vi "基础23.vi"() -> ()   [LabVIEW 2014]
panel:
  out "簇 2":cluster{"数组":dbl[], "数组 2":dbl[]}
  in  "布尔":bool
  in  "簇":cluster{"数组":dbl[], "数组 2":dbl[]}
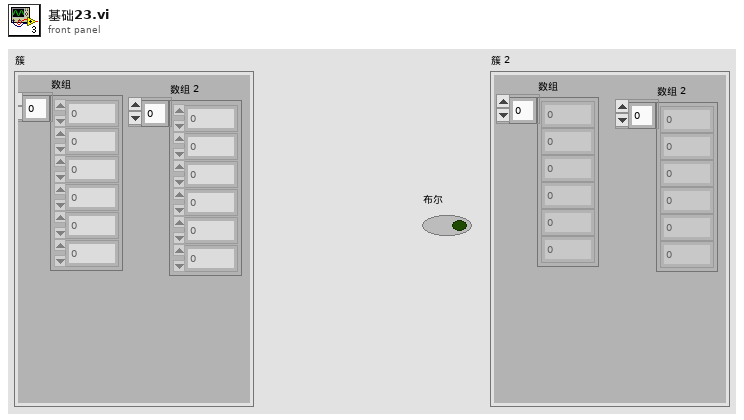
[diagram p1: front panel]
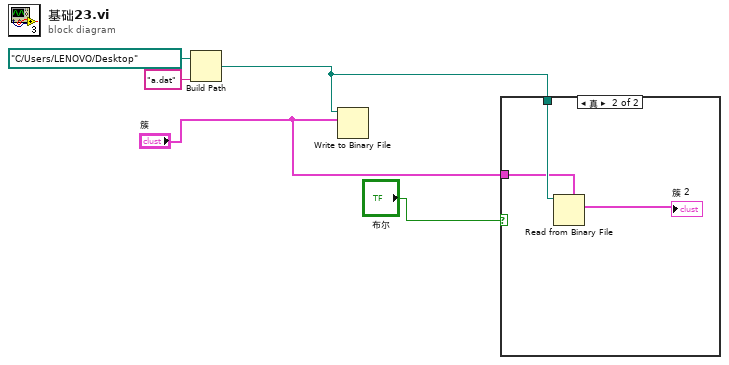
[diagram p0: block diagram]
diagram:
  n1 = Build Path(base path=path "C:/Users/LENOVO/Desktop" ("基路径"), name or relative path="a.dat" ("名称或相对路径")) -> (appended path=w2:path)
  n2 = Write to Binary File(file (use dialog)=w2, data="簇") -> ()  [unwired: 4 in, 3 out]
  n3 = case shown="真" "布尔" {
    tunnel: w2 -> [_ w8]
    tunnel: "簇" -> [_ w7]
    frame False {
    }
    frame True {
      n4 = Read from Binary File(5:w7, 11:w8) -> (2:→"簇 2":cluster{"数组":dbl[], "数组 2":dbl[]})  [unwired: 4 in, 3 out]
    }
  }
